vi "cblas ztrmv.vi"(0 "A":T5, 1 "x":cdb[](array[numeric]), 5 "order":T4=101 items=["CblasRowMajor"=101, "CblasColMajor"=102], 6 "transA":T3=111 items=["CblasNoTrans"=111, "CblasTrans"=112, "CblasConjTrans "=113], 7 "uplo":T1=121 items=["CblasUpper"=121, "CblasLower"=122], 8 "lda":i32, 10 "incx":i32=1, 11 "n":i32=-1, 12 "diag":T2=131 items=["CblasNonUnit"=131, "CblasUnit"=132]) -> (14 "ztrmv":cdb[](array[numeric]), 19 "error":i32)   [LabVIEW 2017, in "NI_AALBLAS.lvlib"]
doc: "Operates on matrix <B>A</B> using the operation you select in <B>operation A</B> and multiplies the result by vector <B>X</B>."
uses:
  NI_AALBLAS.lvlib
  ComplexMatrix.ctl
  Order.ctl
  Operation_Transpose.ctl
  Diag.ctl
  UpLo.ctl
  lvblas.dll
  NI_Matrix.lvlib
panel:
  # "void cblas_ztrmv(order, uplo, transA, diag, n, *A, lda, *x, incx)"
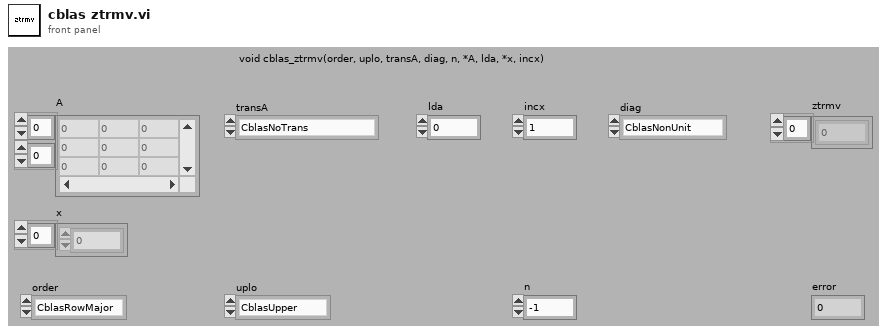
[diagram p1: front panel]
types:
  T1 = typedef "NI_AALBLAS.lvlib/UpLo.ctl" = i32
  T2 = typedef "NI_AALBLAS.lvlib/Diag.ctl" = i32
  T3 = typedef "NI_AALBLAS.lvlib/Operation_Transpose.ctl" = i32
  T4 = typedef "NI_AALBLAS.lvlib/Order.ctl" = i32
  T5 = typedef "NI_Matrix.lvlib/ComplexMatrix.ctl" = cdb[][]
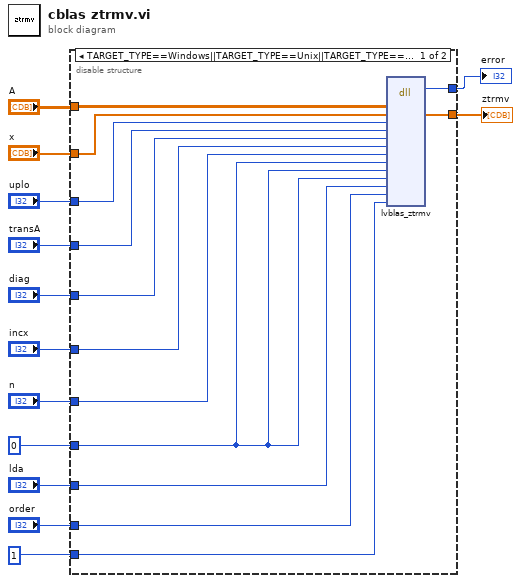
[diagram p0: block diagram]
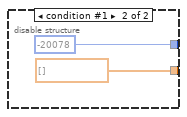
[diagram p2: hidden frame]
diagram:
  n1 = disable-structure shown="TARGET_TYPE==Windows||TARGET_TYPE==Unix||TARGET_TYPE==Mac||TARGET_TYPE==RT" {
    disable-tunnel: "x" -> [w26 _]
    disable-tunnel: "A" -> [w25 _]
    disable-tunnel: [w24 -20078 ("error")] -> w3
    disable-tunnel: 0 -> [w19 _]
    disable-tunnel: "lda" -> [w18 _]
    disable-tunnel: [w23 cdb[] [] ("y")] -> w4
    disable-tunnel: "transA" -> [w16 _]
    disable-tunnel: "uplo" -> [w17 _]
    disable-tunnel: "diag" -> [w22 _]
    disable-tunnel: "incx" -> [w21 _]
    disable-tunnel: "n" -> [w20 _]
    disable-tunnel: "order" -> [w15 _]
    disable-tunnel: 1 -> [w14 _]
    frame condition #0 (active) {
      n2 = dll-call lib="C:/Program Files/National Instruments/LabVIEW 2017/resource/lvblas.*" fn="lvblas_ztrmv" ("CBLAS.dll:MtrxxVectH")("a"=w25, "x"=w26, "uplo"=w17, "OpA"=w16, "diag"=w22, "IncX"=w21, "n"=w20, "startARow"=w19, "startACol"=w19, "startX"=w19, "lda"=w18, "order"=w15, "check"=w14) -> ("error"=w24:i32, "x"=w23:cdb[])  [unwired: 15 in, 2 out]
    }
    frame condition #1 {
    }
  }
  "error" <- w3
  "ztrmv" <- w4
